vi "Auto State Machine.vi"   [LabVIEW 2013]
uses:
  typedefs/fg_typedef.ctl
  typedefs/State Machine/singleUseSubstate.ctl
  typedefs/DevRef Type.ctl
  typedefs/State Machine/subStates.ctl
  typedefs/Vision/vision enable.ctl
panel:
  # "A State Machine to Handle One or Two Ball Autonomous"
types:
  T1 = typedef "fg_typedef.ctl" = enum16{"Get", "Set"}
  T2 = typedef "subStates.ctl" = enum16{"null", "wait", "driver control", "auto", "manual override", "hold position", "rotate", "pickup", "pass", "recover pass", "load", "goto shoot", "shoot high goal", "shoot low goal", "cancel arm", "cancel shooter", "end", "test"}
  T3 = typedef "singleUseSubstate.ctl" = enum16{"null", "wait", "shift high", "shift low", "extend shooter", "retract shooter", "latch", "unlatch", "end"}
  T4 = typedef "vision enable.ctl" = enum16{"Enable", "Disable", "Stop"}
  T5 = typedef "DevRef Type.ctl" = enum16{"Shooter Solenoid", "Latch Solenoid", "Right Up Sensor", "Right Down Sensor", "Hold Sensor", "Arm Encoder"}
  T6 = typedef "WPI_EncoderDevRef.ctl" = cluster{"DevStatus":errorcluster, "EncoderIndex":T7, "CounterIndex":T8, "DistancePerCount":dbl, "Decoding Type":T9}
  T7 = typedef "FPGA_EncoderIdx.ctl" = enum8{"Enc 0", "Enc 1", "Enc 2", "Enc 3", "Invalid"}
  T8 = typedef "FPGA_CounterCtrSystemIndex.ctl" = enum8{"Ctr 0", "Ctr 1", "Ctr 2", "Ctr 3", "Ctr 4", "Ctr 5", "Ctr 6", "Ctr 7", "Invalid"}
  T9 = typedef "WPI_EncoderType.ctl" = enum16{"1x", "2x", "4x"}
  T10 = typedef "WPI_DigitalInputDevRef.ctl" = cluster{"DevStatus":errorcluster, "DIO Channel":T11, "Digital Module":T12}
  T11 = typedef "FPGA_DIOChannel.ctl" = enum8{"DIO 1", "DIO 2", "DIO 3", "DIO 4", "DIO 5", "DIO 6", "DIO 7", "DIO 8", "DIO 9", "DIO 10", "DIO 11", "DIO 12", "DIO 13", "DIO 14", "Invalid"}
  T12 = typedef "FPGA_TypedefDigitalModule.ctl" = enum16{"Digital Module 1", "Digital Module 2"}
  T13 = typedef "vision data.ctl" = cluster{"x":dbl, "y":dbl, "area":dbl, "width":dbl, "height":dbl, "Hot Goal Present?":bool, "distance":dbl}
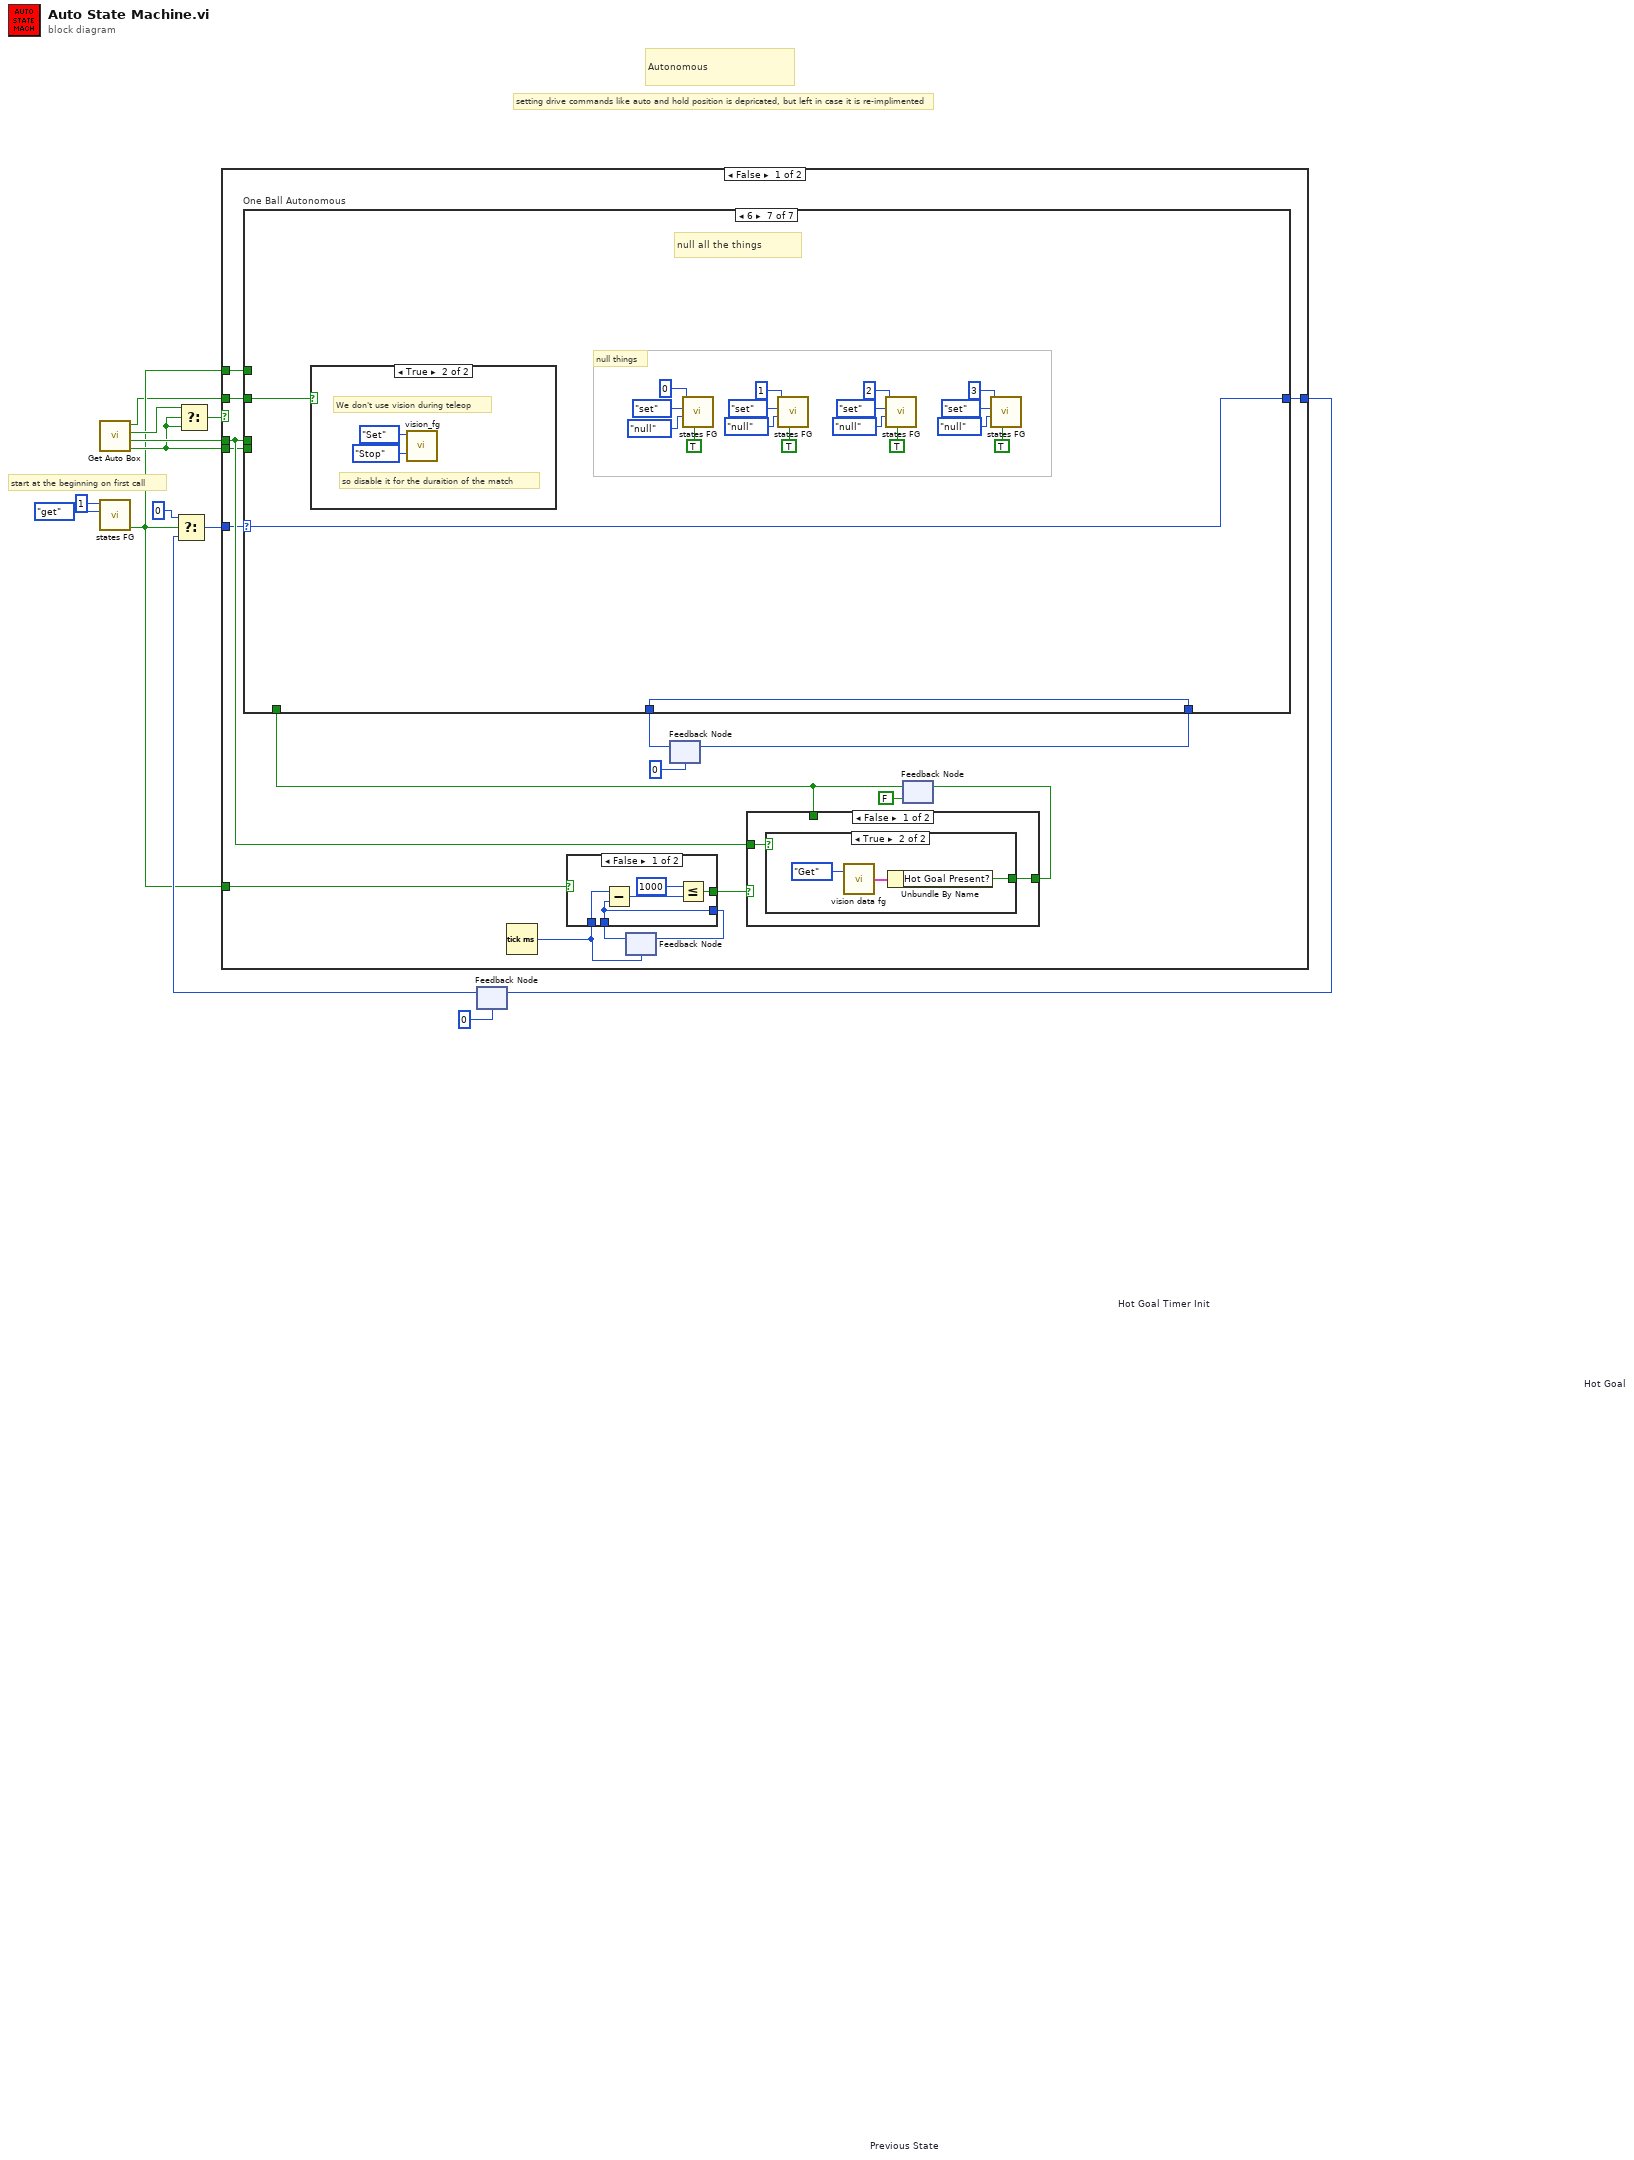
[diagram p0: block diagram]
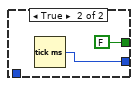
[diagram p2: hidden frame]
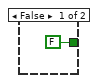
[diagram p3: hidden frame]
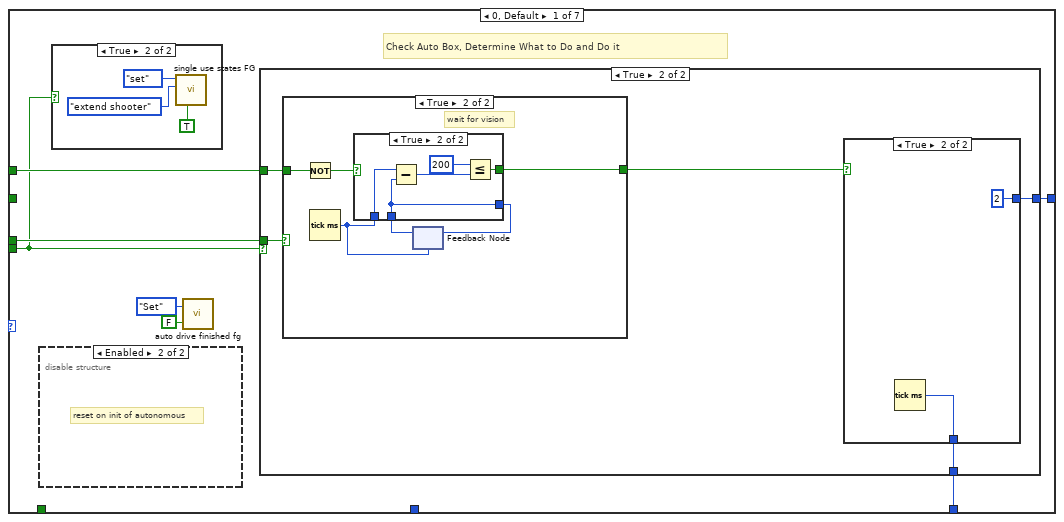
[diagram p5: hidden frame]
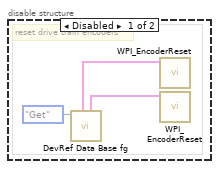
[diagram p6: hidden frame]
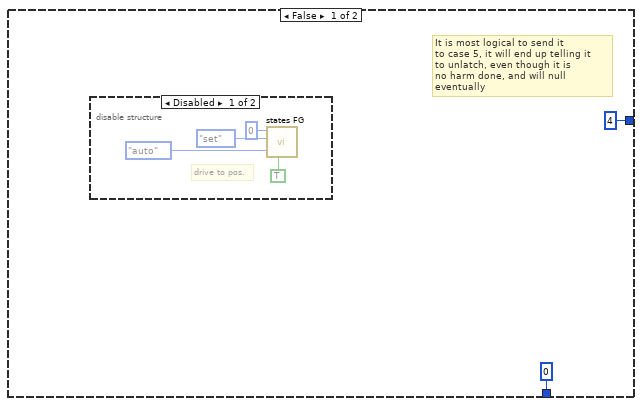
[diagram p7: hidden frame]
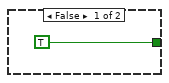
[diagram p9: hidden frame]
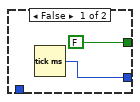
[diagram p10: hidden frame]
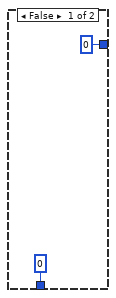
[diagram p11: hidden frame]
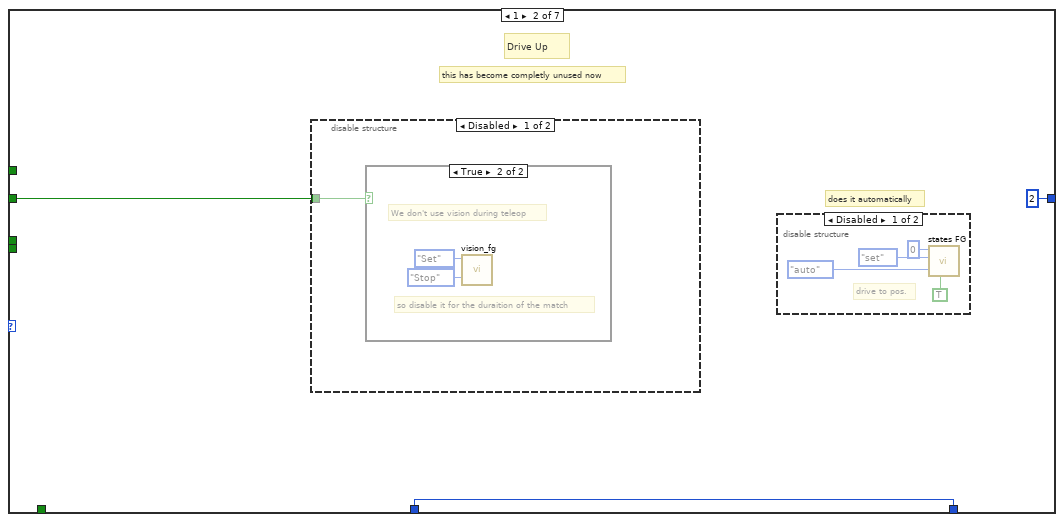
[diagram p13: hidden frame]
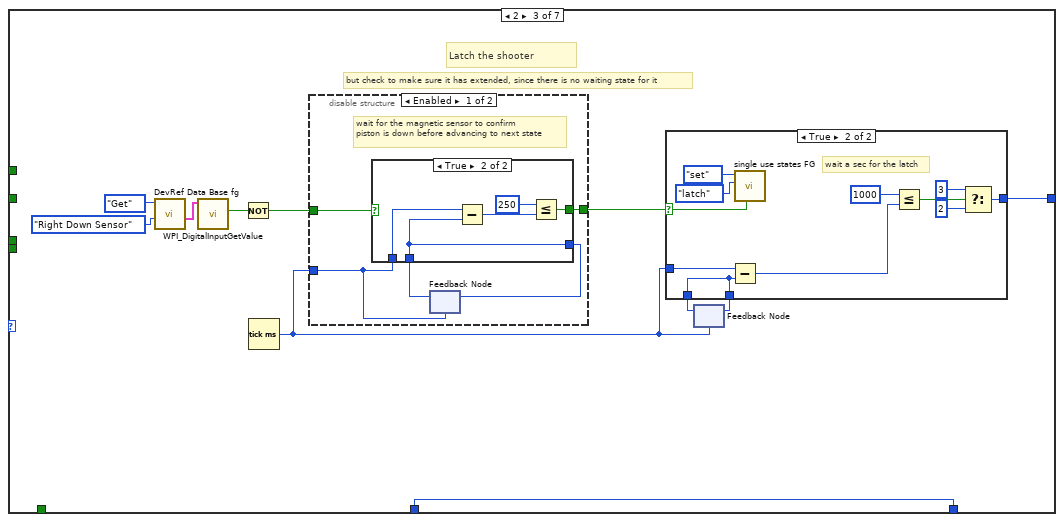
[diagram p17: hidden frame]
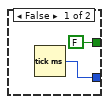
[diagram p18: hidden frame]
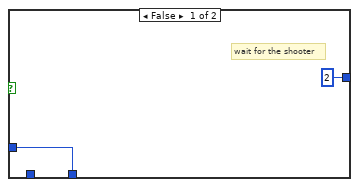
[diagram p20: hidden frame]
diagram:
  # "setting drive commands like auto and hold position is depricated, but left in case it is re-implimented"
  # "start at the beginning on first call"
  # "Autonomous"
  n1 = call "Get Auto Box.vi"() -> ("Shoot During Autonomous?"=w3:bool, "Use Hot Goal?"=w6:bool, "2 Ball Autonomous?"=w4:bool, "Disable Vison After Auto?"=w1:bool)
  n2 = call "states FG.vi"("menu (get)"=enum16{"set", "get"}."get", "Loop ID"=1) -> ("first call?"=w2:bool)  [unwired: 6 in, 3 out]
  n3 = Select(t=w4, s=w3, f=w3) -> (s? t:f=w5:bool)
  n4 = feedback #1 "Previous State"(u8 0) -> (w9:u8)
  n5 = Select(t=u8 0, s=w2, f=w9) -> (s? t:f=w11:u8)
  n6 = case shown="False" w5 {
    tunnel: w11 -> [w29 w226]
    tunnel: [w28 w219] -> w7
    tunnel: w2 -> [w26 w215]
    tunnel: w3 -> [w25 _]
    tunnel: w6 -> [w30 _]
    tunnel: w2 -> [w17 w223]
    tunnel: w1 -> [w23 _]
    frame False {
      n7 = Tick Count (ms)() -> (millisecond timer value=w15:u32)
      n8 = feedback #2(w15) -> (w20:u32)
      n9 = case shown="False" w17 {
        tunnel: [w32 w37] -> w19
        tunnel: w20 -> [w32 _]
        tunnel: [w33 FALSE] -> w18
        tunnel: w15 -> [w31 _]
        frame False {
          n10 = Subtract(x=w31, y=w32) -> (x-y=w35:u32)
          n11 = Less Or Equal?(x=u32 1000, y=w35) -> (x <= y?=w33:bool)
        }
        frame True {
          n12 = Tick Count (ms)() -> (millisecond timer value=w37:u32)
        }
      }
      n13 = feedback-in #2(w19) -> ()
      n14 = feedback #3 "Hot Goal Timer Init"(u32 0 ("millisecond timer value")) -> (w16:u32)
      n15 = feedback #4 "Hot Goal"(FALSE ("Hot Goal Present?")) -> (w14:bool)
      n16 = case "One Ball Autonomous" shown="6" w29 {
        selector: w29 -> [_ _ _ _ w153 _ w212]
        tunnel: [w51 u8 2 ("t") w103 u8 4 ("t") w151 u8 6 ("t") w212] -> w28
        tunnel: w16 -> [_ w89 w97 w134 w141 w187 w195]
        tunnel: w26 -> [w50 _ _ _ _ _ _]
        tunnel: w25 -> [w48 _ _ _ w144 _ _]
        tunnel: w30 -> [w49 _ _ _ _ _ _]
        tunnel: [w47 w89 w97 w134 w141 w187 w195] -> w24
        tunnel: w23 -> [_ w87 _ _ _ _ w194]
        tunnel: w14 -> [_ _ _ _ w143 _ _]
        frame 0, Default {
          # "Check Auto Box, Determine What to Do and Do it"
          n17 = disable-structure shown="Enabled" {
            frame Disabled {
              # "reset drive train encoders"
              n18 = call "DevRef Data Base fg.vi"("Menu"=fg_typedef."Get") -> ("right drive encoder"=w52:T6, "left drive encoder"=w53:T6)  [unwired: 2 in, 7 out]
              n19 = call <vilib>:"WPI_EncoderReset.vi"("EncoderDevRef"=w53) -> ()  [unwired: 9 in, 2 out]
              n20 = call <vilib>:"WPI_EncoderReset.vi"("EncoderDevRef"=w52) -> ()  [unwired: 9 in, 2 out]
            }
            frame Enabled {
              # "reset on init of autonomous"
            }
          }
          n21 = case shown="True" w48 {
            frame False {
            }
            frame True {
              n22 = call "single use states FG.vi"("exit in"=TRUE, "substate"=singleUseSubstate."extend shooter", "menu (get)"=enum16{"set", "get"}."set") -> ()  [unwired: 5 in, 4 out]
            }
          }
          n23 = call "auto drive finished fg.vi"("Done?"=FALSE, "Menu"=fg_typedef."Set") -> ()  [unwired: 1 out]
          n24 = case shown="True" w48 {
            tunnel: [u8 4 ("f") w65] -> w51
            tunnel: w50 -> [_ w64]
            tunnel: w49 -> [_ w62]
            tunnel: [u32 0 ("millisecond timer value") w61] -> w47
            frame False {
              # "It is most logical to send it\nto case 5, it will end up telling it\nto unlatch, even though it is\nno harm done, and will null eventually"
              n25 = disable-structure shown="Disabled" {
                frame Disabled {
                  # "drive to pos."
                  n26 = call "states FG.vi"("exit in"=TRUE, "subState in"=subStates."auto", "menu (get)"=enum16{"set", "get"}."set", "Loop ID"=0) -> ()  [unwired: 4 in, 4 out]
                }
                frame Enabled {
                }
              }
            }
            frame True {
              n27 = case shown="True" w62 {
                tunnel: w64 -> [_ w72]
                tunnel: [TRUE w71] -> w63
                frame False {
                }
                frame True {
                  # "wait for vision"
                  n28 = Not(x=w72) -> (.not. x?=w67:bool)
                  n29 = Tick Count (ms)() -> (millisecond timer value=w70:u32)
                  n30 = feedback #5(w70) -> (w68:u32)
                  n31 = case shown="True" w67 {
                    tunnel: w70 -> [_ w77]
                    tunnel: [w74 w75] -> w69
                    tunnel: w68 -> [_ w75]
                    tunnel: [FALSE w76] -> w71
                    frame False {
                      n32 = Tick Count (ms)() -> (millisecond timer value=w74:u32)
                    }
                    frame True {
                      n33 = Subtract(x=w77, y=w75) -> (x-y=w79:u32)
                      n34 = Less Or Equal?(x=u32 200, y=w79) -> (x <= y?=w76:bool)
                    }
                  }
                  n35 = feedback-in #5(w69) -> ()
                }
              }
              n36 = case shown="True" w63 {
                tunnel: [u8 0 ("f") u8 2 ("f")] -> w65
                tunnel: [u32 0 ("millisecond timer value") w82] -> w61
                frame False {
                }
                frame True {
                  n37 = Tick Count (ms)() -> (millisecond timer value=w82:u32)
                }
              }
            }
          }
        }
        frame 1 {
          # "this has become completly unused now"
          # "does it automatically"
          # "Drive Up"
          n38 = disable-structure shown="Disabled" {
            disable-tunnel: w87 -> [w90 _]
            frame Disabled {
              n39 = case shown="True" w90 {
                frame False {
                }
                frame True {
                  # "so disable it for the duraition of the match"
                  # "We don't use vision during teleop"
                  n40 = call "vision_fg.vi"("Action"=vision_enable."Stop", "Menu"=fg_typedef."Set" ("Enum")) -> ()  [unwired: 1 in, 2 out]
                }
              }
            }
            frame Enabled {
              # "moved to end"
            }
          }
          n41 = disable-structure shown="Disabled" {
            frame Disabled {
              # "drive to pos."
              n42 = call "states FG.vi"("exit in"=TRUE, "subState in"=subStates."auto", "menu (get)"=enum16{"set", "get"}."set", "Loop ID"=0) -> ()  [unwired: 4 in, 4 out]
            }
            frame Enabled {
            }
          }
        }
        frame 2 {
          # "but check to make sure it has extended, since there is no waiting state for it"
          # "Latch the shooter"
          n43 = call "DevRef Data Base fg.vi"("DevRef to Get"=DevRef_Type."Right Down Sensor", "Menu"=fg_typedef."Get") -> ("Selected Sensor"=w107:T10)  [unwired: 1 in, 8 out]
          n44 = call <vilib>:"WPI_DigitalInputGetValue.vi"("DigitalInputDevRef"=w107) -> ("Value"=w106:bool)  [unwired: 8 in, 2 out]
          n45 = Not(x=w106) -> (.not. x?=w100:bool)
          n46 = Tick Count (ms)() -> (millisecond timer value=w99:u32)
          n47 = disable-structure shown="Enabled" {
            disable-tunnel: w100 -> [w112 w120]
            disable-tunnel: [w109 w120] -> w98
            disable-tunnel: w99 -> [w108 _]
            frame Enabled {
              # "wait for the magnetic sensor to confirm \npiston is down before advancing to next state"
              n48 = feedback #6(w108) -> (w110:u32)
              n49 = case shown="True" w112 {
                tunnel: w108 -> [_ w117]
                tunnel: [w114 w115] -> w111
                tunnel: w110 -> [_ w115]
                tunnel: [FALSE w116] -> w109
                frame False {
                  n50 = Tick Count (ms)() -> (millisecond timer value=w114:u32)
                }
                frame True {
                  n51 = Subtract(x=w117, y=w115) -> (x-y=w119:u32)
                  n52 = Less Or Equal?(x=u32 250, y=w119) -> (x <= y?=w116:bool)
                }
              }
              n53 = feedback-in #6(w111) -> ()
            }
            frame Disabled {
            }
          }
          n54 = feedback #7(w99) -> (w104:u32)
          n55 = case shown="True" w98 {
            selector: w98 -> [_ w129]
            tunnel: [w121 w131] -> w105
            tunnel: w104 -> [_ w131]
            tunnel: w99 -> [w121 w130]
            tunnel: [u8 2 ("f") w124] -> w103
            frame False {
              # "wait for the shooter"
            }
            frame True {
              # "wait a sec for the latch"
              n56 = Subtract(x=w130, y=w131) -> (x-y=w126:u32)
              n57 = call "single use states FG.vi"("exit in"=w129, "substate"=singleUseSubstate."latch", "menu (get)"=enum16{"set", "get"}."set") -> ()  [unwired: 5 in, 4 out]
              n58 = Less Or Equal?(x=u32 1000, y=w126) -> (x <= y?=w123:bool)
              n59 = Select(t=u8 3, s=w123, f=u8 2) -> (s? t:f=w124:u8)
            }
          }
          n60 = feedback-in #7(w105) -> ()
        }
        frame 3 {
          # "just go on, nothing to\nwait for"
          # "retract shooter"
          n61 = call "single use states FG.vi"("exit in"=TRUE, "substate"=singleUseSubstate."retract shooter", "menu (get)"=enum16{"set", "get"}."set") -> ()  [unwired: 5 in, 4 out]
        }
        frame 4 {
          # "depends on if shooting"
          # "at setpoint?"
          n62 = case shown="False" w143 {
            tunnel: w141 -> [w170 w176]
            tunnel: [w169 w175] -> w142
            frame True {
              # "get it first cycle after 3.5 seconds"
              n63 = Tick Count (ms)() -> (millisecond timer value=w171:u32)
              n64 = Subtract(x=w171, y=w170) -> (x-y=w173:u32)
              n65 = disable-structure shown="Disabled" {
                disable-tunnel: [_ FALSE ("Done")] -> w167
                frame Disabled {
                }
                frame Enabled {
                }
              }
              n66 = Less Or Equal?(x=u32 3500, y=w173) -> (x <= y?=w168:bool)
              n67 = Or(x=w168, y=w167) -> (x .or. y?=w169:bool)
            }
            frame False {
              # "wait 5.25 seconds for hot goal to switch"
              n68 = Tick Count (ms)() -> (millisecond timer value=w177:u32)
              n69 = Subtract(x=w177, y=w176) -> (x-y=w179:u32)
              n70 = Less Or Equal?(x=u32 5250, y=w179) -> (x <= y?=w175:bool)
            }
          }
          n71 = disable-structure shown="Enabled" {
            disable-tunnel: w141 -> [w156 _]
            frame Disabled {
              n72 = Tick Count (ms)() -> (millisecond timer value=w159:u32)
              n73 = Subtract(x=w159, y=w156) -> (x-y=w157:u32)
              n74 = Less Or Equal?(x=u32 4100, y=w157) -> (x <= y?=w155:bool)
              n75 = disable-structure shown="Enabled" {
                disable-tunnel: w155 -> [w161 _]
                disable-tunnel: fg_typedef."Set" ("Menu") -> [w160 _]
                frame Enabled {
                  n76 = case shown="True" w161 {
                    selector: w161 -> [_ w163]
                    tunnel: w160 -> [_ w162]
                    frame False {
                    }
                    frame True {
                      n77 = call "auto drive finished fg.vi"("Done?"=w163, "Menu"=w162) -> ()  [unwired: 1 out]
                      n78 = call "states FG.vi"("exit in"=w163, "subState in"=subStates."null" ("y"), "menu (get)"=enum16{"set", "get"}."set", "Loop ID"=0) -> ()  [unwired: 4 in, 4 out]
                    }
                  }
                }
                frame Disabled {
                }
              }
            }
            frame Enabled {
            }
          }
          n79 = call "DevRef Data Base fg.vi"("DevRef to Get"=DevRef_Type."Right Up Sensor", "Menu"=fg_typedef."Get") -> ("Selected Sensor"=w150:T10)  [unwired: 1 in, 8 out]
          n80 = call <vilib>:"WPI_DigitalInputGetValue.vi"("DigitalInputDevRef"=w150) -> ("Value"=w149:bool)  [unwired: 8 in, 2 out]
          n81 = Not(x=w149) -> (.not. x?=w146:bool)
          n82 = case shown="True" w146 {
            frame False {
            }
            frame True {
              # "incase we have problems,\nlet drivers trigger shoot after auto\nsince it is infact safe to shoot now"
              n83 = call "safe shoot error.vi"("Can Shoot Safely?"=TRUE, "Menu"=fg_typedef."Set") -> ()  [unwired: 1 out]
            }
          }
          n84 = call "auto drive finished fg.vi"("Menu"=fg_typedef."Get") -> ("Done"=w139:bool)  [unwired: 1 in]
          n85 = case shown="False" w144 {
            tunnel: w142 -> [_ w184]
            tunnel: w146 -> [_ w183]
            tunnel: w139 -> [w180 w182]
            tunnel: [w180 w181] -> w145
            frame False {
            }
            frame True {
              n86 = Compound Arithmetic op=AND(w184, w183, w182) -> (w181:bool)
            }
          }
          n87 = Select(t=u8 5, s=w145, f=w153) -> (s? t:f=w151:u8)
        }
        frame 5 {
          w190 = FALSE ("Can Shoot Safely?")
          w189 = fg_typedef."Set" ("Menu")
          # "unlatch shooter"
          # "SHOOT!!!"
          n88 = call "safe shoot error.vi"("Can Shoot Safely?"=w190, "Menu"=w189) -> ()  [unwired: 1 out]
          n89 = call "auto drive finished fg.vi"("Done?"=w190, "Menu"=w189) -> ()  [unwired: 1 out]
          n90 = call "single use states FG.vi"("exit in"=TRUE, "substate"=singleUseSubstate."unlatch", "menu (get)"=enum16{"set", "get"}."set") -> ()  [unwired: 5 in, 4 out]
        }
        frame 6 {
          # "null things"
          # "null all the things"
          n91 = case shown="True" w194 {
            frame False {
            }
            frame True {
              # "so disable it for the duraition of the match"
              # "We don't use vision during teleop"
              n92 = call "vision_fg.vi"("Action"=vision_enable."Stop", "Menu"=fg_typedef."Set" ("Enum")) -> ()  [unwired: 1 in, 2 out]
            }
          }
          n93 = call "states FG.vi"("exit in"=TRUE, "subState in"=subStates."null", "menu (get)"=enum16{"set", "get"}."set", "Loop ID"=0) -> ()  [unwired: 4 in, 4 out]
          n94 = call "states FG.vi"("exit in"=TRUE, "subState in"=subStates."null", "menu (get)"=enum16{"set", "get"}."set", "Loop ID"=1) -> ()  [unwired: 4 in, 4 out]
          n95 = call "states FG.vi"("exit in"=TRUE, "subState in"=subStates."null", "menu (get)"=enum16{"set", "get"}."set", "Loop ID"=2) -> ()  [unwired: 4 in, 4 out]
          n96 = call "states FG.vi"("exit in"=TRUE, "subState in"=subStates."null", "menu (get)"=enum16{"set", "get"}."set", "Loop ID"=3) -> ()  [unwired: 4 in, 4 out]
        }
      }
      n97 = feedback-in #3(w24) -> ()
      n98 = case shown="False" w18 {
        tunnel: [w39 w44] -> w21
        tunnel: w14 -> [_ w44]
        tunnel: w30 -> [w38 _]
        frame False {
          n99 = case shown="True" w38 {
            tunnel: [FALSE ("Hot Goal Present?") w43] -> w39
            frame False {
            }
            frame True {
              n100 = call "vision data fg.vi"("Menu"=fg_typedef."Get") -> ("Output"=w42:T13)  [unwired: 1 in]
              n101 = Unbundle By Name(w42) -> ("Hot Goal Present?"=w43:bool)
            }
          }
        }
        frame True {
        }
      }
      n102 = feedback-in #4(w21) -> ()
    }
    frame True {
      n103 = feedback #8 "Wait Timer Init"(u32 0 ("millisecond timer value")) -> (w216:u32)
      n104 = case "Two Ball Autonomous" shown="0, Default" w226 {
        selector: w226 -> [_ w303 _ w322 _ w356 _ _ w377 w415 _ w433]
        tunnel: [u8 1 ("t") w305 u8 3 ("t") w319 u8 5 ("t") w358 u8 7 ("t") u8 8 ("t") w378 w414 u8 11 ("t") w433] -> w219
        tunnel: [_ _ w313 w320 _ _ _ _ _ _ _ _] -> w217
        tunnel: w216 -> [_ _ _ w321 _ _ _ _ _ _ _ _]
        tunnel: w215 -> [w284 _ _ _ _ _ _ _ _ _ _ _]
        frame 0, Default {
          # "full reverse is belts in"
          # "belts on"
          # "up setpoint"
          # "put arm out"
          # "Arm Up, Belts In"
          # "reset drive train encoders"
          n105 = case shown="True" w284 {
            frame False {
            }
            frame True {
              # "so disable it for the duraition of the match"
              # "We don't use vision during teleop"
              n106 = call "vision_fg.vi"("Action"=vision_enable."Stop", "Menu"=fg_typedef."Set" ("Enum")) -> ()  [unwired: 1 in, 2 out]
            }
          }
          n107 = call "auto drive finished fg.vi"("Done?"=FALSE, "Menu"=fg_typedef."Set") -> ()  [unwired: 1 out]
          n108 = call "Arm Setpoint FG.vi"("Setpoint In"=55.0, "Menu"=fg_typedef."Set") -> ()  [unwired: 1 out]
          n109 = call "states FG.vi"("exit in"=TRUE, "subState in"=subStates."auto", "menu (get)"=enum16{"set", "get"}."set", "Loop ID"=3) -> ()  [unwired: 4 in, 4 out]
          n110 = call "Belt Speed FG.vi"("Speed In"=-1.0 ("Setpoint In"), "Menu"=fg_typedef."Set") -> ()  [unwired: 1 out]
          n111 = call "states FG.vi"("exit in"=TRUE, "subState in"=subStates."auto", "menu (get)"=enum16{"set", "get"}."set", "Loop ID"=2) -> ()  [unwired: 4 in, 4 out]
          n112 = call "DevRef Data Base fg.vi"("Menu"=fg_typedef."Get") -> ("right drive encoder"=w298:T6, "left drive encoder"=w299:T6)  [unwired: 2 in, 7 out]
          n113 = call <vilib>:"WPI_EncoderReset.vi"("EncoderDevRef"=w299) -> ()  [unwired: 9 in, 2 out]
          n114 = call <vilib>:"WPI_EncoderReset.vi"("EncoderDevRef"=w298) -> ()  [unwired: 9 in, 2 out]
        }
        frame 1 {
          # "Wait for Arm"
          n115 = call "DevRef Data Base fg.vi"("DevRef to Get"=DevRef_Type."Arm Encoder", "Menu"=fg_typedef."Get") -> ("Selected Encoder"=w312:T6)  [unwired: 1 in, 8 out]
          n116 = call <vilib>:"WPI_EncoderGet.vi"("EncoderDevRef"=w312) -> ("Distance"=w311:dbl)  [unwired: 5 in, 5 out]
          n117 = In Range and Coerce(upper limit=55.0, x=w311, lower limit=45.0) -> (In Range?=w304:bool)  [unwired: 1 out]
          n118 = Select(t=u8 2, s=w304, f=w303) -> (s? t:f=w305:u8)
        }
        frame 2 {
          # "drive to reverse position"
          n119 = Tick Count (ms)() -> (millisecond timer value=w313:u32)
          n120 = call "states FG.vi"("exit in"=TRUE, "subState in"=subStates."auto", "menu (get)"=enum16{"set", "get"}."set", "Loop ID"=0) -> ()  [unwired: 4 in, 4 out]
        }
        frame 3 {
          # "Wait for Ball"
          n121 = disable-structure shown="Enabled" {
            disable-tunnel: w322 -> [w324 w333]
            disable-tunnel: w321 -> [_ w335]
            disable-tunnel: [_ w335] -> w320
            disable-tunnel: [w323 w331] -> w319
            frame Disabled {
              n122 = call "DevRef Data Base fg.vi"("DevRef to Get"=DevRef_Type."Hold Sensor", "Menu"=fg_typedef."Get") -> ("Selected Sensor"=w328:T10)  [unwired: 1 in, 8 out]
              n123 = call <vilib>:"WPI_DigitalInputGetValue.vi"("DigitalInputDevRef"=w328) -> ("Value"=w330:bool)  [unwired: 8 in, 2 out]
              n124 = Not(x=w330) -> (.not. x?=w329:bool)
              n125 = Select(t=u8 4, s=w329, f=w324) -> (s? t:f=w323:u8)
            }
            frame Enabled {
              n126 = Tick Count (ms)() -> (millisecond timer value=w338:u32)
              n127 = Subtract(x=w338, y=w335) -> (x-y=w337:u32)
              n128 = Less Or Equal?(x=u32 1000, y=w337) -> (x <= y?=w334:bool)
              n129 = Select(t=u8 4, s=w334, f=w333) -> (s? t:f=w331:u8)
            }
          }
        }
        frame 4 {
          # "drive to forward position"
          # "arm rests on ball"
          # "reset fg"
          # "reset fg"
          # "Belts Off, Arm Hold Ball"
          n130 = call "states FG.vi"("exit in"=TRUE, "subState in"=subStates."auto", "menu (get)"=enum16{"set", "get"}."set", "Loop ID"=0) -> ()  [unwired: 4 in, 4 out]
          n131 = call "Belt Speed FG.vi"("Speed In"=0.0 ("Setpoint In"), "Menu"=fg_typedef."Set") -> ()  [unwired: 1 out]
          n132 = call "states FG.vi"("exit in"=TRUE, "subState in"=subStates."null", "menu (get)"=enum16{"set", "get"}."set", "Loop ID"=3) -> ()  [unwired: 4 in, 4 out]
          n133 = call "states FG.vi"("exit in"=TRUE, "subState in"=subStates."null", "menu (get)"=enum16{"set", "get"}."set", "Loop ID"=2) -> ()  [unwired: 4 in, 4 out]
          n134 = call "Arm Setpoint FG.vi"("Setpoint In"=0.0, "Menu"=fg_typedef."Set") -> ()  [unwired: 1 out]
        }
        frame 5 {
          w362 = fg_typedef."Get" ("Menu")
          # "Ready to Shoot 1st Ball?"
          n135 = call "safe shoot error.vi"("Menu"=w362) -> ("Can Shoot Safely?"=w361:bool)  [unwired: 1 in]
          n136 = call "auto drive finished fg.vi"("Menu"=w362) -> ("Done"=w360:bool)  [unwired: 1 in]
          n137 = And(x=w361, y=w360) -> (x .and. y?=w357:bool)
          n138 = Select(t=u8 6, s=w357, f=w356) -> (s? t:f=w358:u8)
        }
        frame 6 {
          w365 = FALSE ("Can Shoot Safely?")
          w364 = fg_typedef."Set" ("Menu")
          # "unlatch shooter"
          # "stop driving"
          n139 = call "states FG.vi"("exit in"=TRUE, "subState in"=subStates."hold position", "menu (get)"=enum16{"set", "get"}."set", "Loop ID"=0) -> ()  [unwired: 4 in, 4 out]
          n140 = call "safe shoot error.vi"("Can Shoot Safely?"=w365, "Menu"=w364) -> ()  [unwired: 1 out]
          n141 = call "auto drive finished fg.vi"("Done?"=w365, "Menu"=w364) -> ()  [unwired: 1 out]
          n142 = call "single use states FG.vi"("exit in"=TRUE, "substate"=singleUseSubstate."unlatch", "menu (get)"=enum16{"set", "get"}."set") -> ()  [unwired: 5 in, 4 out]
        }
        frame 7 {
          # "Cock again"
          # "extend shooter"
          n143 = call "single use states FG.vi"("exit in"=TRUE, "substate"=singleUseSubstate."extend shooter", "menu (get)"=enum16{"set", "get"}."set") -> ()  [unwired: 5 in, 4 out]
        }
        frame 8 {
          # "Wait to Latch Shooter, Then Latch"
          n144 = call "DevRef Data Base fg.vi"("DevRef to Get"=DevRef_Type."Right Down Sensor", "Menu"=fg_typedef."Get") -> ("Selected Sensor"=w380:T10)  [unwired: 1 in, 8 out]
          n145 = call <vilib>:"WPI_DigitalInputGetValue.vi"("DigitalInputDevRef"=w380) -> ("Value"=w379:bool)  [unwired: 8 in, 2 out]
          n146 = Tick Count (ms)() -> (millisecond timer value=w387:u32)
          n147 = Not(x=w379) -> (.not. x?=w383:bool)
          n148 = disable-structure shown="Enabled" {
            disable-tunnel: w383 -> [w405 w413]
            disable-tunnel: [w402 w413] -> w386
            disable-tunnel: w387 -> [w401 _]
            frame Enabled {
              # "wait for the magnetic sensor to confirm \npiston is down before advancing to next state"
              n149 = feedback #9(w401) -> (w403:u32)
              n150 = case shown="True" w405 {
                tunnel: w401 -> [_ w410]
                tunnel: [w407 w408] -> w404
                tunnel: w403 -> [_ w408]
                tunnel: [FALSE w409] -> w402
                frame False {
                  n151 = Tick Count (ms)() -> (millisecond timer value=w407:u32)
                }
                frame True {
                  n152 = Subtract(x=w410, y=w408) -> (x-y=w412:u32)
                  n153 = Less Or Equal?(x=u32 250, y=w412) -> (x <= y?=w409:bool)
                }
              }
              n154 = feedback-in #9(w404) -> ()
            }
            frame Disabled {
            }
          }
          n155 = feedback #10(w387) -> (w385:u32)
          n156 = case shown="True" w386 {
            selector: w386 -> [_ w396]
            tunnel: [w389 w398] -> w384
            tunnel: w385 -> [_ w398]
            tunnel: w387 -> [w389 w397]
            tunnel: [w388 w392] -> w378
            tunnel: w377 -> [w388 w390]
            frame False {
              # "wait for the shooter"
            }
            frame True {
              # "wait a sec for the latch"
              n157 = Subtract(x=w397, y=w398) -> (x-y=w393:u32)
              n158 = call "single use states FG.vi"("exit in"=w396, "substate"=singleUseSubstate."latch", "menu (get)"=enum16{"set", "get"}."set") -> ()  [unwired: 5 in, 4 out]
              n159 = Less Or Equal?(x=u32 1000, y=w393) -> (x <= y?=w391:bool)
              n160 = Select(t=u8 9, s=w391, f=w390) -> (s? t:f=w392:u8)
            }
          }
          n161 = feedback-in #10(w384) -> ()
        }
        frame 9 {
          # "Retract Shooter"
          # "retract shooter"
          n162 = call "single use states FG.vi"("exit in"=TRUE, "substate"=singleUseSubstate."retract shooter", "menu (get)"=enum16{"set", "get"}."set") -> ()  [unwired: 5 in, 4 out]
          n163 = call "DevRef Data Base fg.vi"("DevRef to Get"=DevRef_Type."Right Up Sensor", "Menu"=fg_typedef."Get") -> ("Selected Sensor"=w416:T10)  [unwired: 1 in, 8 out]
          n164 = call <vilib>:"WPI_DigitalInputGetValue.vi"("DigitalInputDevRef"=w416) -> ("Value"=w417:bool)  [unwired: 8 in, 2 out]
          n165 = Not(x=w417) -> (.not. x?=w421:bool)
          n166 = case shown="True" w421 {
            frame False {
            }
            frame True {
              # "incase we have problems,\nlet drivers trigger shoot after auto\nsince it is infact safe to shoot now"
              n167 = call "safe shoot error.vi"("Can Shoot Safely?"=TRUE, "Menu"=fg_typedef."Set") -> ()  [unwired: 1 out]
            }
          }
          n168 = Select(t=u8 10, s=w421, f=w415) -> (s? t:f=w414:u8)
        }
        frame 10 {
          w429 = FALSE ("Can Shoot Safely?")
          w428 = fg_typedef."Set" ("Menu")
          # "unlatch shooter"
          # "Shoot Second Ball"
          n169 = call "safe shoot error.vi"("Can Shoot Safely?"=w429, "Menu"=w428) -> ()  [unwired: 1 out]
          n170 = call "auto drive finished fg.vi"("Done?"=w429, "Menu"=w428) -> ()  [unwired: 1 out]
          n171 = call "single use states FG.vi"("exit in"=TRUE, "substate"=singleUseSubstate."unlatch", "menu (get)"=enum16{"set", "get"}."set") -> ()  [unwired: 5 in, 4 out]
        }
        frame 11 {
          # "Null Everything"
          # "null things"
          n172 = call "states FG.vi"("exit in"=TRUE, "subState in"=subStates."null", "menu (get)"=enum16{"set", "get"}."set", "Loop ID"=0) -> ()  [unwired: 4 in, 4 out]
          n173 = call "states FG.vi"("exit in"=TRUE, "subState in"=subStates."null", "menu (get)"=enum16{"set", "get"}."set", "Loop ID"=1) -> ()  [unwired: 4 in, 4 out]
          n174 = call "states FG.vi"("exit in"=TRUE, "subState in"=subStates."null", "menu (get)"=enum16{"set", "get"}."set", "Loop ID"=2) -> ()  [unwired: 4 in, 4 out]
          n175 = call "states FG.vi"("exit in"=TRUE, "subState in"=subStates."null", "menu (get)"=enum16{"set", "get"}."set", "Loop ID"=3) -> ()  [unwired: 4 in, 4 out]
        }
      }
      n176 = feedback-in #8(w217) -> ()
      n177 = feedback #11 "Previous State"(u8 0) -> (w221:u8)
      n178 = Select(t=u8 0, s=w223, f=w221) -> (s? t:f=w224:u8)
      n179 = case "Parallel Initial Pneumatics" shown="0, Default" w224 {
        selector: w224 -> [_ w231 w278 w281]
        tunnel: [u8 1 ("t") w234 w269 w281] -> w220
        frame 0, Default {
          # "Cock Shooter for Pre-Loaded Ball"
          # "extend shooter"
          n180 = call "single use states FG.vi"("exit in"=TRUE, "substate"=singleUseSubstate."extend shooter", "menu (get)"=enum16{"set", "get"}."set") -> ()  [unwired: 5 in, 4 out]
        }
        frame 1 {
          # "Wait to Latch Shooter, Then Latch"
          n181 = call "DevRef Data Base fg.vi"("DevRef to Get"=DevRef_Type."Right Down Sensor", "Menu"=fg_typedef."Get") -> ("Selected Sensor"=w240:T10)  [unwired: 1 in, 8 out]
          n182 = call <vilib>:"WPI_DigitalInputGetValue.vi"("DigitalInputDevRef"=w240) -> ("Value"=w241:bool)  [unwired: 8 in, 2 out]
          n183 = Tick Count (ms)() -> (millisecond timer value=w232:u32)
          n184 = Not(x=w241) -> (.not. x?=w237:bool)
          n185 = disable-structure shown="Enabled" {
            disable-tunnel: w237 -> [w259 w267]
            disable-tunnel: [w256 w267] -> w233
            disable-tunnel: w232 -> [w255 _]
            frame Enabled {
              # "wait for the magnetic sensor to confirm \npiston is down before advancing to next state"
              n186 = feedback #12(w255) -> (w257:u32)
              n187 = case shown="True" w259 {
                tunnel: w255 -> [_ w264]
                tunnel: [w261 w262] -> w258
                tunnel: w257 -> [_ w262]
                tunnel: [FALSE w263] -> w256
                frame False {
                  n188 = Tick Count (ms)() -> (millisecond timer value=w261:u32)
                }
                frame True {
                  n189 = Subtract(x=w264, y=w262) -> (x-y=w266:u32)
                  n190 = Less Or Equal?(x=u32 250, y=w266) -> (x <= y?=w263:bool)
                }
              }
              n191 = feedback-in #12(w258) -> ()
            }
            frame Disabled {
            }
          }
          n192 = feedback #13(w232) -> (w235:u32)
          n193 = case shown="True" w233 {
            selector: w233 -> [_ w250]
            tunnel: [w243 w252] -> w236
            tunnel: w235 -> [_ w252]
            tunnel: w232 -> [w243 w251]
            tunnel: [w242 w246] -> w234
            tunnel: w231 -> [w242 w244]
            frame False {
              # "wait for the shooter"
            }
            frame True {
              # "wait a sec for the latch"
              n194 = Subtract(x=w251, y=w252) -> (x-y=w247:u32)
              n195 = call "single use states FG.vi"("exit in"=w250, "substate"=singleUseSubstate."latch", "menu (get)"=enum16{"set", "get"}."set") -> ()  [unwired: 5 in, 4 out]
              n196 = Less Or Equal?(x=u32 1000, y=w247) -> (x <= y?=w245:bool)
              n197 = Select(t=u8 2, s=w245, f=w244) -> (s? t:f=w246:u8)
            }
          }
          n198 = feedback-in #13(w236) -> ()
        }
        frame 2 {
          # "retract shooter"
          # "Retract Shooter"
          n199 = call "single use states FG.vi"("exit in"=TRUE, "substate"=singleUseSubstate."retract shooter", "menu (get)"=enum16{"set", "get"}."set") -> ()  [unwired: 5 in, 4 out]
          n200 = call "DevRef Data Base fg.vi"("DevRef to Get"=DevRef_Type."Right Up Sensor", "Menu"=fg_typedef."Get") -> ("Selected Sensor"=w274:T10)  [unwired: 1 in, 8 out]
          n201 = call <vilib>:"WPI_DigitalInputGetValue.vi"("DigitalInputDevRef"=w274) -> ("Value"=w273:bool)  [unwired: 8 in, 2 out]
          n202 = Not(x=w273) -> (.not. x?=w268:bool)
          n203 = case shown="True" w268 {
            frame False {
            }
            frame True {
              # "incase we have problems,\nlet drivers trigger shoot after auto\nsince it is infact safe to shoot now"
              n204 = call "safe shoot error.vi"("Can Shoot Safely?"=TRUE, "Menu"=fg_typedef."Set") -> ()  [unwired: 1 out]
            }
          }
          n205 = Select(t=u8 3, s=w268, f=w278) -> (s? t:f=w269:u8)
        }
        frame 3 {
        }
      }
      n206 = feedback-in #11(w220) -> ()
    }
  }
  n207 = feedback-in #1(w7) -> ()
